vi "RenderDiff.vi"(8 "error in (no error)":errorcluster, 11 "DiffVI in":refnum<class "DiffVI.lvclass">) -> (0 "error out":errorcluster, 3 "DiffVI out":refnum<class "DiffVI.lvclass">)   [LabVIEW 2020, in "DiffVI.lvclass"]
uses:
  DiffVI.lvclass
  DiffVI.lvclass/DiffVI.ctl
  Modules/Screenshots/VIDiffScreenshots.lvlib
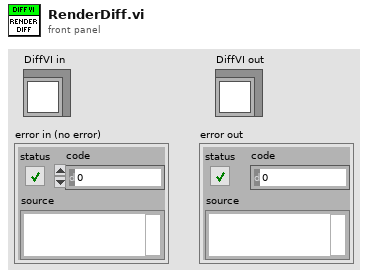
[diagram p1: front panel]
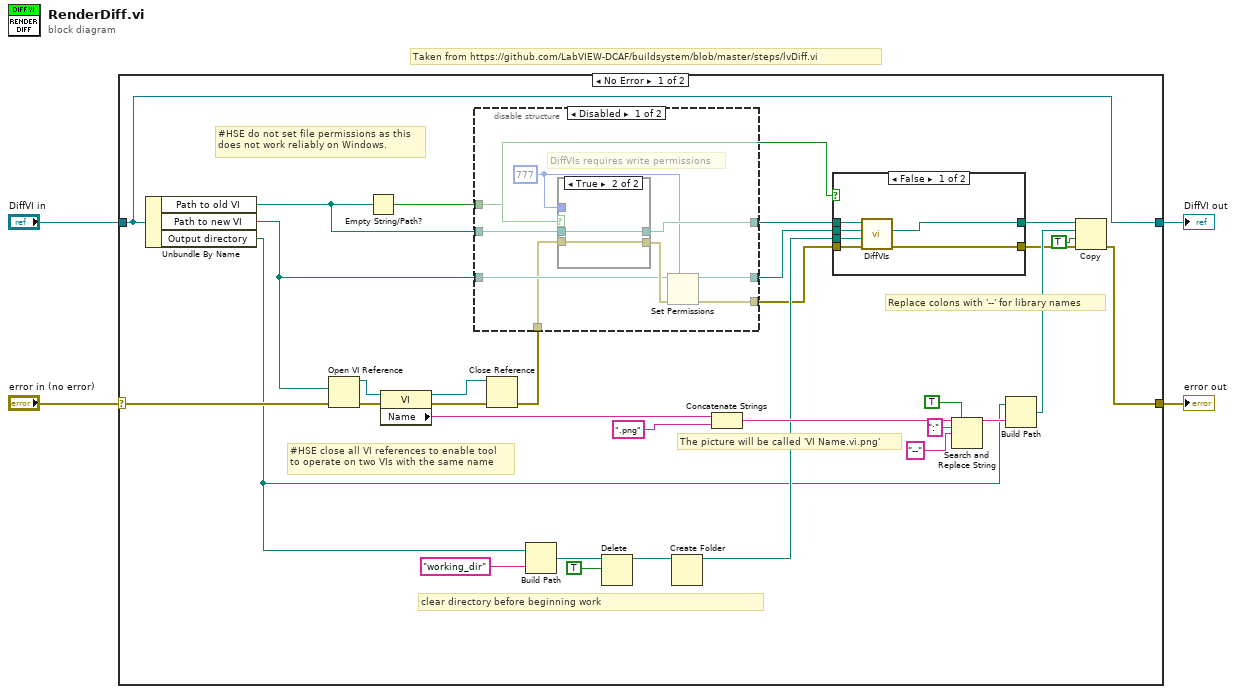
[diagram p0: block diagram]
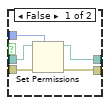
[diagram p2: hidden frame]
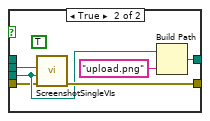
[diagram p4: hidden frame]
diagram:
  # "Taken from https://github.com/LabVIEW-DCAF/buildsystem/blob/master/steps/lvDiff.vi"
  n1 = case shown="No Error" "error in (no error)" {
    selector: "error in (no error)" -> [w35 w68]
    tunnel: [w21 w68] -> w3
    tunnel: "DiffVI in" -> [w12 w67]
    tunnel: [w12 w67] -> w1
    frame No Error {
      # "#HSE do not set file permissions as this\ndoes not work reliably on Windows."
      # "#HSE close all VI references to enable tool \nto operate on two VIs with the same name"
      # "Replace colons with '--' for library names"
      # "clear directory before beginning work"
      # "The picture will be called 'VI Name.vi.png'"
      n2 = Unbundle By Name(w12) -> ("Path to old VI"=w8:path, "Path to new VI"=w10:path, "Output directory"=w11:path)
      n3 = Open VI Reference(vi path=w10, error in (no error)=w35) -> (vi reference=w23:refnum<vi>, error out=w24:errorcluster)  [unwired: 4 in]
      n4 = Empty String/Path?(string/path=w8) -> (empty?=w9:bool)
      n5 = property class="VI"(reference=w23, error in=w24) -> (reference out=w7:refnum<vi>, error out=w6:errorcluster, "Name"=w25:string)
      n6 = Close Reference(reference=w7, error in (no error)=w6) -> (error out=w5:errorcluster)
      n7 = disable-structure shown="Disabled" {
        disable-tunnel: [w44 w54] -> w33
        disable-tunnel: [w41 w53] -> w14
        disable-tunnel: [w40 w52] -> w13
        disable-tunnel: w10 -> [w39 w53]
        disable-tunnel: w9 -> [w38 _]
        disable-tunnel: w8 -> [w37 w54]
        disable-tunnel: w5 -> [w36 w52]
        frame Disabled {
          w43 = i16 777 ("permissions")
          # "DiffVIs requires write permissions"
          n8 = case shown="True" w38 {
            tunnel: w37 -> [w49 w50]
            tunnel: [w48 w51] -> w42
            tunnel: w43 -> [w47 _]
            tunnel: w36 -> [w46 w51]
            tunnel: [w45 w50] -> w44
            frame False {
              n9 = Set Permissions(7:w47, 8:w46, 11:w49) -> (0:w48:errorcluster, 3:w45:path)  [unwired: 2 in]
            }
            frame True {
            }
          }
          n10 = Set Permissions(7:w43, 8:w42, 11:w39) -> (0:w40:errorcluster, 3:w41:path)  [unwired: 2 in]
        }
        frame Enabled {
        }
      }
      n11 = Build Path(base path=w11, name or relative path="working_dir") -> (appended path=w26:path)
      n12 = Delete(path (use dialog)=w26, entire hierarchy (F)=TRUE) -> (deleted path=w27:path)  [unwired: 3 in, 2 out]
      n13 = Create Folder(path (use dialog)=w27) -> (created path=w16:path)  [unwired: 2 in, 2 out]
      n14 = Concatenate Strings(w25, ".png" ("string")) -> (w32:string)
      n15 = case shown="False" w9 {
        tunnel: w13 -> [w60 w62]
        tunnel: w14 -> [w59 w61]
        tunnel: [w58 w66] -> w15
        tunnel: w16 -> [w57 w63]
        tunnel: [w56 w64] -> w17
        tunnel: w33 -> [w55 _]
        frame False {
          n16 = call "DiffVIs.vi"("error in"=w60, "Picture Save Location"=w57, "New VI Path"=w59, "Old VI Path"=w55) -> ("error out"=w56:errorcluster, "diff file"=w58:path)  [unwired: 6 in]
        }
        frame True {
          (unwired) TRUE ("Take Scrshots All In")
          n17 = call "ScreenshotSingleVIs.vi"("error in"=w62, "Picture Save Location"=w63, "New VI Path"=w61) -> ("error out"=w64:errorcluster)  [unwired: 8 in]
          n18 = Build Path(base path=w63, name or relative path="upload.png") -> (appended path=w66:path)
        }
      }
      n19 = Search and Replace String(replace all?=TRUE ("replace all? (F)"), input string=w32, search string=":", replace string="--" ("replace string (\"\")")) -> (result string=w29:string)  [unwired: 4 in, 3 out]
      n20 = Build Path(base path=w11, name or relative path=w29) -> (appended path=w20:path)
      n21 = Copy(8:w17, 9:TRUE ("overwrite (F)"), 10:w20, 11:w15) -> (0:w21:errorcluster)  [unwired: 1 in, 2 out]
    }
    frame Error {
    }
  }
  "error out" <- w3
  "DiffVI out" <- w1
